vi "ClearHardwareTasks_RT.vi"(1 "Task cluster":T1={"inbits"=8, "outbits"=38, "Counter"="Counter", "Inbits"="Inbits", "Outbits"="Outbits", "Fast AO"=["FastAO_1", "FastAO_2", "FastAO_3"], "Errors"={"status"=FALSE, "code"=0, "source"=""}}) -> (0 "Errors":errorcluster)   [LabVIEW 2018]
uses:
  Target/Tasks_RT.ctl
panel:
  # "Tasks and errors"
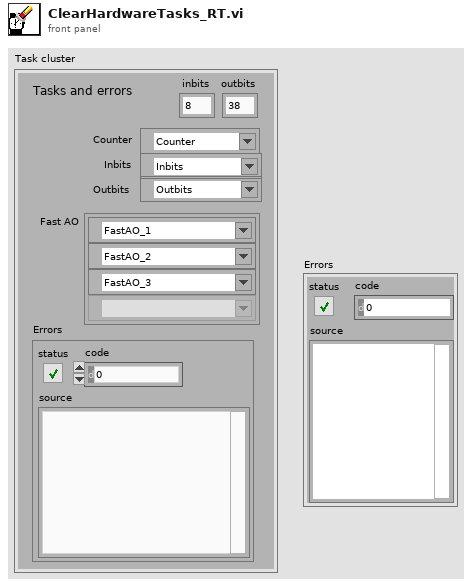
[diagram p1: front panel]
types:
  T1 = typedef "Tasks_RT.ctl" = cluster{"inbits":i32, "outbits":i32, "Counter":refnum<k21>, "Inbits":refnum<k21>, "Outbits":refnum<k21>, "Fast AO":refnum<k21>[], "Errors":errorcluster}
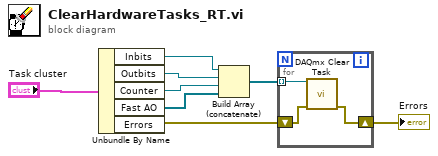
[diagram p0: block diagram]
diagram:
  n1 = Unbundle By Name("Task cluster") -> ("Inbits"=w5:refnum<k21>, "Outbits"=w6:refnum<k21>, "Counter"=w8:refnum<k21>, "Fast AO"=w2:refnum<k21>[], "Errors"=w1:errorcluster)
  n2 = Build Array (concatenate)(w5, w6, w8, w2) -> (w4:refnum<k21>[])
  n3 = for {
    shift-right: [w10] -> w3
    shift-left: w1 -> [w11]
    tunnel: w4 -> [w9] mode=indexing
    n4 = call <vilib>:"DAQmx Clear Task.vi"("task in"=w9, "error in"=w11) -> ("error out"=w10:errorcluster)  [unwired: 13 in]
  }
  "Errors" <- w3
